vi "TCP Server.vi"() -> ()   [LabVIEW 2020]
uses:
  <vilib>/addons/_JKI.lib/_JKI_lib_TCP_Server.llb/TCP Server Public Connections Info Cluster.ctl
  <userlib>/_NEVSTOP/Communicable State Machine(CSM)/_Support/Typedef/_CSM_GlobalLog_MSG.ctl
  <userlib>/_NEVSTOP/Communicable State Machine(CSM)/_Support/Typedef/_CSM_Response Source Message.ctl
  <userlib>/_NEVSTOP/Communicable State Machine(CSM)/_Support/Typedef/_CSM_GlobalLog_MSG_TYPE.ctl
  <userlib>/_NEVSTOP/Communicable State Machine(CSM)/_Support/Priority Queue/Priority Queue.lvclass/Priority Queue.ctl
  931d4ba7-b454-410e-88bd-402e2cce69a9.vi
  <vilib>/Utility/error.llb/Clear Errors.vi
  <userlib>/_NEVSTOP/Communicable State Machine(CSM)/addons/INI-Static-Variable-Support/_Support/Supported Type.vi
  931d4ba7-b454-410e-88bd-402e2cce69a9.vi/b09b9099-6be0-413b-8afc-4908471460c3.vi
  <userlib>/_NEVSTOP/Communicable State Machine(CSM)/_Support/Process/CSMP-Sync Call.vi
  <userlib>/_NEVSTOP/Communicable State Machine(CSM)/Utility/uuid.vi
  <userlib>/_NEVSTOP/Communicable State Machine(CSM)/Utility/Trim Both Whitespace.vi
  <userlib>/_NEVSTOP/Communicable State Machine(CSM)/_Support/CSMQ/_CSMObj-Message Check.vi
  <userlib>/_NEVSTOP/Communicable State Machine(CSM)/_Support/CSMQ/_CSMObj-Enqueue Cross-Module Message.vi
  <userlib>/_NEVSTOP/Communicable State Machine(CSM)/_Support/CSMQ/_CSMOFGV Get.vi
  <userlib>/_NEVSTOP/Communicable State Machine(CSM)/_Support/Priority Queue/Enqueue Element.vi
  <userlib>/_NEVSTOP/Communicable State Machine(CSM)/addons/INI-Static-Variable-Support/_Support/global-csm-ini-db-change-flag.vi
  <vilib>/Utility/Data Type/Get Type Information.vi
  <userlib>/_NEVSTOP/Communicable State Machine(CSM)/addons/API-String-Arugments-Support/_Support/Data To SingleElementsArray_csm.vi
  <userlib>/_NEVSTOP/Communicable State Machine(CSM)/addons/API-String-Arugments-Support/_Support/Data To API String Arguments.vi
  <userlib>/_NEVSTOP/Communicable State Machine(CSM)/addons/INI-Static-Variable-Support/_Support/Parse Used Session and Name.vi
  <userlib>/_NEVSTOP/Communicable State Machine(CSM)/addons/INI-Static-Variable-Support/_Support/INI-FGV2.vi
  <userlib>/_NEVSTOP/Communicable State Machine(CSM)/addons/API-String-Arugments-Support/_Support/Convert API String Arguments to Data(variant).vi
  <userlib>/_NEVSTOP/Communicable State Machine(CSM)/addons/API-String-Arugments-Support/_Support/SingleElementsArray To Data_csm.vi
  <userlib>/_NEVSTOP/Communicable State Machine(CSM)/Utility/Build Error Cluster.vi
  <userlib>/_NEVSTOP/Communicable State Machine(CSM)/_Support/CSMQ/_CSMOFGV.vi
  <vilib>/addons/_JKI.lib/_JKI_lib_TCP_Server.llb/JKI TCP Server.lvclass
  <userlib>/_NEVSTOP/Communicable State Machine(CSM)/Communicable State Machine.lvlib
  <userlib>/_NEVSTOP/Communicable State Machine(CSM)/addons/INI-Static-Variable-Support/INI-Static-Variable-Support.lvlib
panel:
  out "String Cache":string
  in  "stop":bool
  out "Connections Info":T1[](array[typedef])
  out "No. of Connections":u32
  out "Time Running":dbl[unit] format="%#.0p"
  in  "Disconnect all clients?":bool
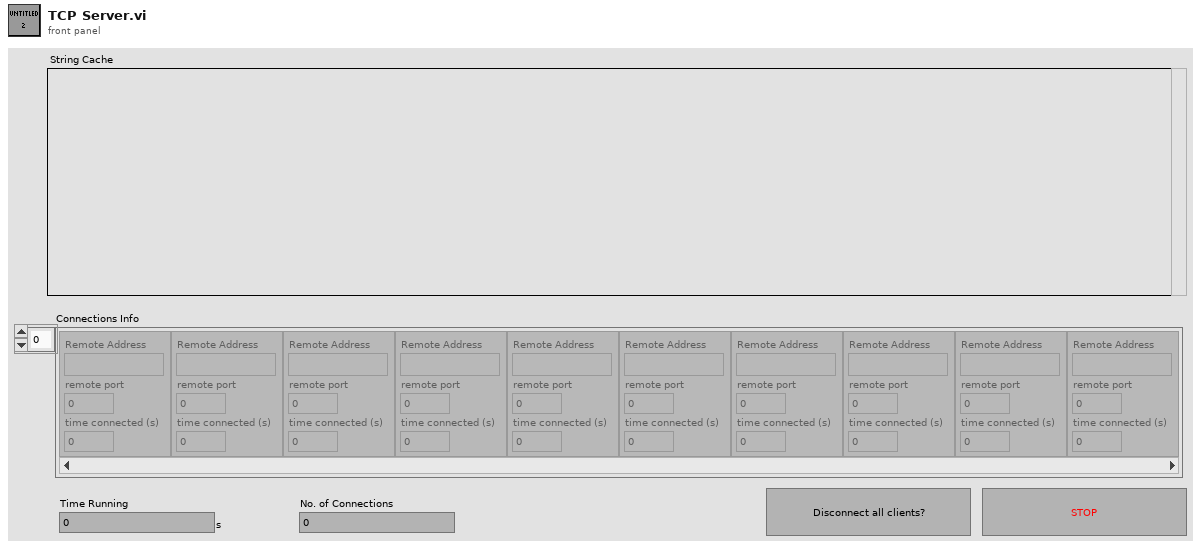
[diagram p1: front panel]
types:
  T1 = typedef "JKI TCP Server.lvclass/TCP Server Public Connections Info Cluster.ctl" = cluster{"Remote Address":string, "remote port":u16, "time connected (s)":dbl}
  T2 = cluster{"Server.Port":u16, "Server.MaxConnections":u32}
  T3 = typedef "Communicable State Machine.lvlib/_CSM_GlobalLog_MSG.ctl" = cluster{"Name(\"\" to use uuid)":string, "Current State":string, "Arguments":string, "Source Message":T4, "Source Module":string, "Complete(T)/Start(F)":bool, "LogType":T5}
  T4 = typedef "Communicable State Machine.lvlib/_CSM_Response Source Message.ctl" = cluster{"‘State":string, "’Arguments":string, "’Error":errorcluster}
  T5 = typedef "Communicable State Machine.lvlib/_CSM_GlobalLog_MSG_TYPE.ctl" = enum16{"User Log", "State Change", "Status", "Interrupt", "Register", "Unregister", "Error Log", "Module Created", "Module Destroyed"}
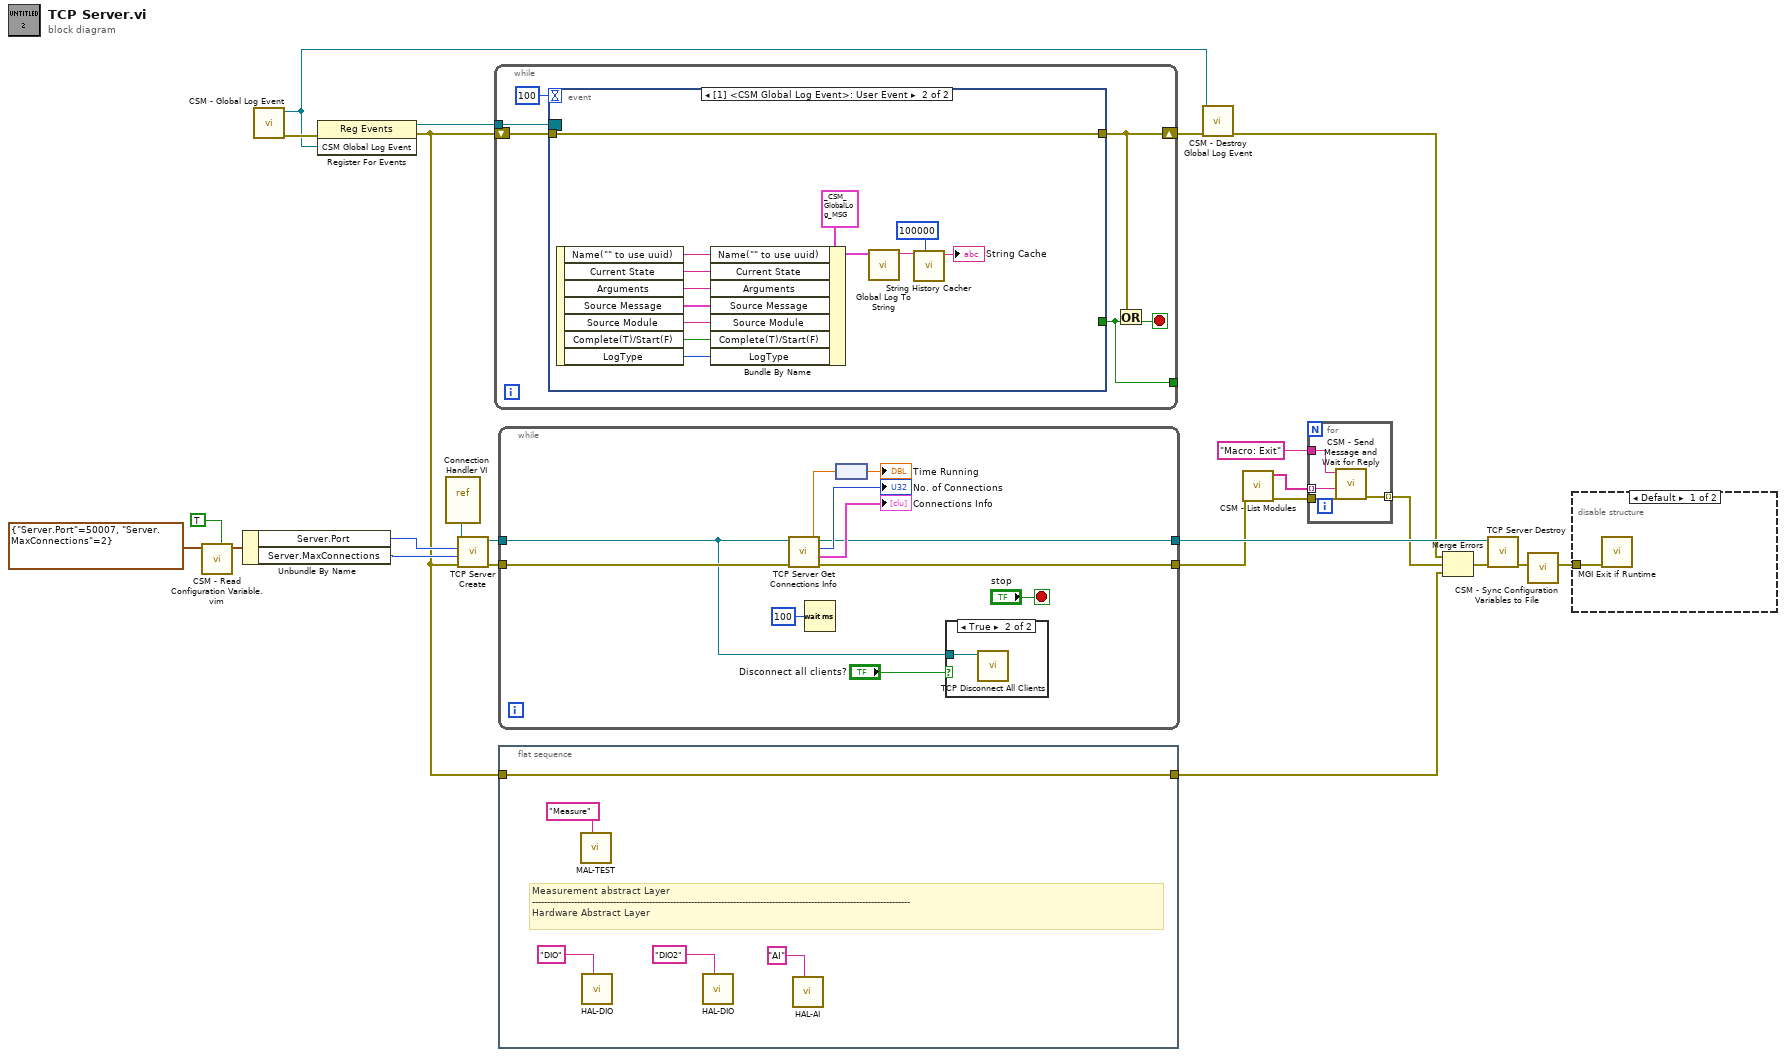
[diagram p0: block diagram]
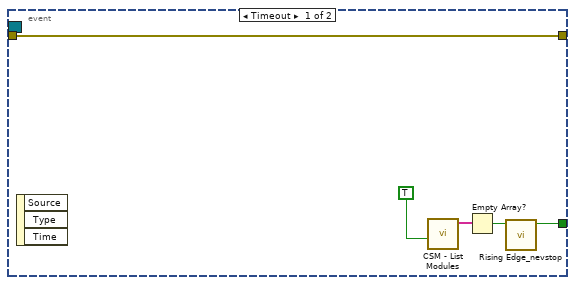
[diagram p3: hidden frame]
diagram:
  n1 = call "CSM - Read Configuration Variable.vim"("Write If not found?(F)"=TRUE, "config prototype(Cluster Prefered)"=T2 {"Server.Port"=50007, "Server.MaxConnections"=2}) -> ("config out"=w19:T2)  [unwired: 6 in, 1 out]
  n2 = Unbundle By Name(w19) -> ("Server.Port"=w18:u16, "Server.MaxConnections"=w17:u32)
  n3 = call <userlib>:"CSM - Global Log Event.vi"() -> ("Error out"=w14:errorcluster, "CSM Global Log Event"=w13:refnum<user-event>)  [unwired: 10 in]
  n4 = register-events(error in=w14, w13) -> (reference out=w16:refnum<event-registration>, error out=w4:errorcluster)  [unwired: 1 in]
  n5 = vi-ref "Connection Handler VI.vi"() -> ("vi reference"=w21:refnum<vi>)
  n6 = call <vilib>:"TCP Server Create.vi"("error in (no error)"=w4, "max connections (0: no limit)"=w17, "port"=w18, "Connection Handler Call-Back VI RefNum"=w21) -> ("error out"=w24:errorcluster, "TCP Server"=w23:refnum<class "JKI TCP Server.lvclass">)  [unwired: 6 in]
  n7 = while {
    tunnel: w16 -> [w30]
    shift-right: [w27] -> w15
    shift-left: w4 -> [w29]
    tunnel: [w26] -> _
    stop <- w28 stop-if-true
    n8 = event shown="[1] <CSM Global Log Event>: User Event" {
      selector: w30 -> [_ _]
      dyn-events: _ -> [_ _]
      timeout: 100 -> [_ _]
      tunnel: w29 -> [w35 w39]
      tunnel: [w35 w39] -> w27
      tunnel: [w31 _] -> w26
      event Timeout {
        n9 = event-data() -> ()  [unwired: 1 in, 3 out]
        n10 = call <userlib>:"CSM - List Modules.vi"("All?"=TRUE) -> ("Module Names"=w34:string[])  [unwired: 9 in, 1 out]
        n11 = Empty Array?(array=w34) -> (empty?=w33:bool)
        n12 = call <userlib>:"Rising Edge_nevstop.vi"("signal"=w33) -> ("rising edge"=w31:bool)  [unwired: 10 in]
      }
      event User Event {
        n13 = event-data() -> ("Name(\"\" to use uuid)"=w48:string, "Current State"=w47:string, "Arguments"=w46:string, "Source Message"=w45:T4, "Source Module"=w44:string, "Complete(T)/Start(F)"=w43:bool, "LogType"=w42:T5)  [unwired: 1 in]
        n14 = Bundle By Name(cluster=T3 {"Name(\"\" to use uuid)"="", "Current State"="", "Arguments"="", "Source Message"={"‘State"="", "’Arguments"="", "’Error"={"status"=FALSE, "code"=0, "source"=""}}, "Source Module"="", "Complete(T)/Start(F)"=FALSE, "LogType"=enum."State Change"} ("Cross CSM Data"), "Name(\"\" to use uuid)"=w48, "Current State"=w47, "Arguments"=w46, "Source Message"=w45, "Source Module"=w44, "Complete(T)/Start(F)"=w43, "LogType"=w42) -> (w40:T3)
        n15 = call <userlib>:"Global Log To String.vi"("Log"=w40) -> ("Log String"=w38:string)  [unwired: 9 in]
        n16 = call <userlib>:"String History Cacher.vi"("length"=100000, "String"=w38) -> ("String Cache"=→"String Cache":string)  [unwired: 9 in]
      }
    }
    n17 = Or(x=w27, y=w26) -> (x .or. y?=w28:bool)
  }
  n18 = while {
    tunnel: w24 -> [w54]
    tunnel: w23 -> [w51]
    tunnel: [w53] -> w22
    tunnel: [w52] -> w9
    stop <- "stop" stop-if-true
    n19 = call <vilib>:"TCP Server Get Connections Info.vi"("error in (no error)"=w54, "TCP Server"=w51) -> ("error out"=w52:errorcluster, "Connections Info"=→"Connections Info":T1[], "Number of Connections"=→"No. of Connections":u32, "TCP Server out"=w53:refnum<class "JKI TCP Server.lvclass">, "time running (s)"=w57:dbl)  [unwired: 5 in]
    n20 = Wait (ms)(milliseconds to wait=u32 100) -> ()  [unwired: 1 out]
    n21 = node(w57) -> (→"Time Running":dbl[unit])
    n22 = case shown="True" "Disconnect all clients?" {
      tunnel: w51 -> [_ w60]
      frame False {
      }
      frame True {
        n23 = call <vilib>:"TCP Disconnect All Clients.vi"("TCP Server"=w60) -> ()  [unwired: 9 in, 2 out]
      }
    }
  }
  n24 = flat-sequence {
    tunnel: w4 -> [w65]
    tunnel: [w65] -> w10
    frame #0 {
      # "Measurement abstract Layer\n------------------------------------------------------------------------------------------------------------------------------\nHardware Abstract Layer"
      n25 = call "MAL-TEST.vi"("Name(\"\" to use uuid)"="Measure" ("Name(\"\" to use uuid)")) -> ()  [unwired: 11 in]
      n26 = call "HAL-DIO.vi"("Name(\"\" to use uuid)"="DIO" ("Name(\"\" to use uuid)")) -> ()  [unwired: 11 in]
      n27 = call "HAL-DIO.vi"("Name(\"\" to use uuid)"="DIO2" ("Name(\"\" to use uuid)")) -> ()  [unwired: 11 in]
      n28 = call "HAL-AI.vi"("Name(\"\" to use uuid)"="AI" ("Name(\"\" to use uuid)")) -> ()  [unwired: 11 in]
    }
  }
  n29 = call <userlib>:"CSM - Destroy Global Log Event.vi"("Error in"=w15, "CSM Global Log Event"=w13) -> ("Error out"=w11:errorcluster)  [unwired: 9 in]
  n30 = call <userlib>:"CSM - List Modules.vi"("Error in"=w9) -> ("Error out"=w8:errorcluster, "Module Names"=w7:string[])  [unwired: 9 in]
  n31 = for {
    tunnel: w8 -> [w69]
    tunnel: w7 -> [w68] mode=indexing
    tunnel: "Macro: Exit" ("State") -> [w67]
    tunnel: [w66] -> w5 mode=indexing
    n32 = call <userlib>:"CSM - Send Message and Wait for Reply.vi"("Error In (no error)"=w69, "Target Module"=w68, "State"=w67) -> ("error out"=w66:errorcluster)  [unwired: 6 in, 2 out]
  }
  n33 = Merge Errors(w11, w5, w10) -> (w12:errorcluster)
  n34 = call <vilib>:"TCP Server Destroy.vi"("error in (no error)"=w12, "TCP Server"=w22) -> ("error out"=w3:errorcluster)  [unwired: 9 in]
  n35 = call <userlib>:"CSM - Sync Configuration Variables to File.vi"("error in (no error)"=w3) -> ("error out"=w2:errorcluster)  [unwired: 8 in]
  n36 = disable-structure "Conditional Disable Structure" shown="Default" {
    disable-tunnel: w2 -> [w70 _]
    frame condition #0 (active) {
      n37 = call <userlib>:"MGI Exit if Runtime.vi"("Error In (Dependency Only)"=w70) -> ()  [unwired: 11 in]
    }
    frame condition #1 {
    }
  }
